vi "SMO.UI.ByRefWithEvents.TestLauncher.vi"() -> ()   [LabVIEW 2013, in "SMO.UI.ByRefWithEvents.lvclass"]
doc: "JKI State Machine Objects (SMO) 1.0.0.5\nJKI - JKI\nCopyright (c) 2016, JKI"
uses:
  SMO.UI.ByRefWithEvents.lvclass
  <vilib>/JKI/JKI SMO/SMO/SMO.lvclass
  <vilib>/JKI/JKI SMO/SMO.UI/SMO.UI.lvclass
panel:
  in  "Send":bool
  in  "Data":string
  out "error out":errorcluster
  in  "Stop":bool
  # "SMO UI Test Launcher"
  # "For instructions on how to use the JKI State Machine Objects, examples and video tutorials, visit:\nhttp://jki.net/state-machine-objects/\n\nJKI State Machine Objects™\nhttp://jki.net/state-machine-objects/\nCopyright (C) 2005-2015, JKI <info@jki.net>\nALL RIGHTS RESERVED"
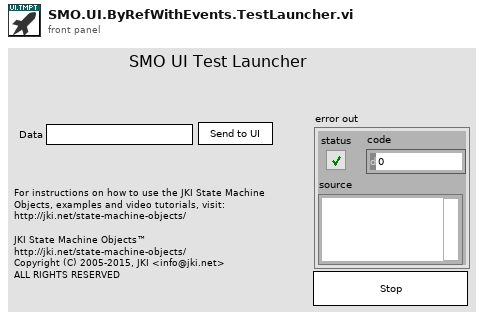
[diagram p1: front panel]
types:
  T1 = typedef "SMO.UI.lvclass/PublicEvents--Cluster.ctl" = cluster{"UI Hidden":refnum<user-event>, "UI State":refnum<user-event>}
  T2 = cluster{"SMO.Template Public Events":refnum<event-registration>, "Event Registration Refnum":refnum<event-registration>}
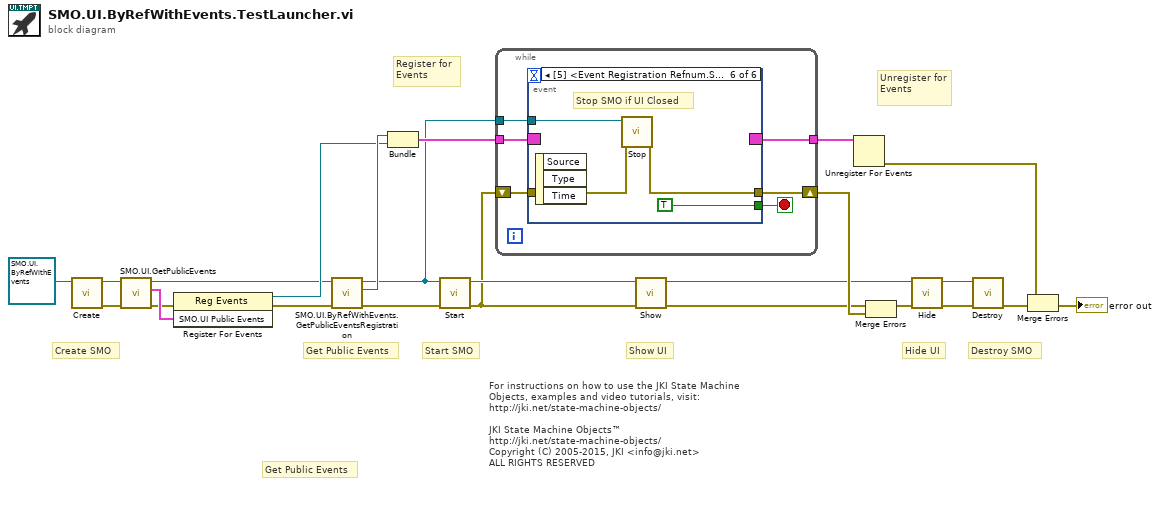
[diagram p0: block diagram]
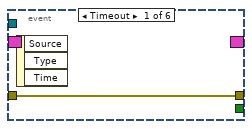
[diagram p2: hidden frame]
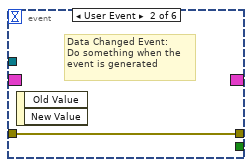
[diagram p3: hidden frame]
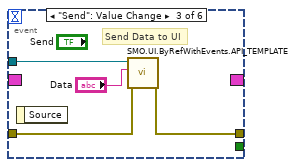
[diagram p4: hidden frame]
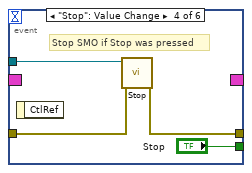
[diagram p5: hidden frame]
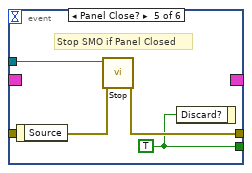
[diagram p6: hidden frame]
diagram:
  # "Get Public Events"
  # "Hide UI"
  # "Show UI"
  # "For instructions on how to use the JKI State Machine Objects, examples and video tutorials, visit:\nhttp://jki.net/state-machine-objects/\n\nJKI State Machine Objects™\nhttp://jki.net/state-machine-objects/\nCopyright (C) 2005-2015, JKI <info@jki.net>\nALL RIGHTS RESERVED"
  # "Get Public Events"
  # "Start SMO"
  # "Destroy SMO"
  # "Create SMO"
  # "Unregister for Events"
  # "Register for Events"
  n1 = call <vilib>:"Create.vi"("SMO"=refnum<class "SMO.UI.ByRefWithEvents.lvclass"> refnum ("SMO.Template.lvclass")) -> ("error out"=w2:errorcluster, "SMO out"=w5:refnum<class "SMO.UI.ByRefWithEvents.lvclass">)  [unwired: 8 in, 1 out]
  n2 = call <vilib>:"SMO.UI.GetPublicEvents.vi"("error in (no error)"=w2, "SMO.UI"=w5) -> ("error out"=w6:errorcluster, "SMO.UI Public Events"=w7:T1, "SMO.UI out"=w3:refnum<class "SMO.UI.ByRefWithEvents.lvclass">)  [unwired: 7 in]
  n3 = register-events(error in=w6, w7) -> (reference out=w4:refnum<event-registration>, error out=w1:errorcluster)  [unwired: 1 in]
  n4 = call "SMO.UI.ByRefWithEvents.GetPublicEventsRegistration.vi"("error in (no error)"=w1, "SMO.UI.ByRefWithEvents"=w3) -> ("error out"=w17:errorcluster, "SMO.Template Public Events"=w16:refnum<event-registration>, "SMO.UI.ByRefWithEvents out"=w15:refnum<class "SMO.UI.ByRefWithEvents.lvclass">)  [unwired: 7 in]
  n5 = Bundle("SMO.Template Public Events"=w16, "Event Registration Refnum"=w4) -> (w23:T2)  [unwired: 1 in]
  n6 = call <vilib>:"Start.vi"("error in (no error)"=w17, "SMO"=w15) -> ("error out"=w13:errorcluster, "SMO out"=w14:refnum<class "SMO.UI.ByRefWithEvents.lvclass">)  [unwired: 8 in]
  n7 = while {
    shift-right: [w29] -> w22
    shift-left: w13 -> [w28]
    tunnel: w23 -> [w27]
    tunnel: [w26] -> w24
    tunnel: w15 -> [w25]
    stop <- w30 stop-if-true
    n8 = event shown="[5] <Event Registration Refnum.SMO.UI Public Events.UI Hidden>: User Event" {
      selector: w27 -> [_ _ _ _ _ _]
      dyn-events: [_ _ _ _ _ _] -> w26
      timeout: _ -> [_ _ _ _ _ _]
      tunnel: [_ _ _ "Stop" w41 TRUE ("OK")] -> w30
      tunnel: w25 -> [_ _ w36 w38 w44 w48]
      tunnel: [w31 w32 w33 w39 w43 w47] -> w29
      tunnel: w28 -> [w31 w32 w34 w37 w42 w46]
      event Timeout {
        n9 = event-data() -> ()  [unwired: 1 in, 3 out]
      }
      event User Event {
        # "Data Changed Event:\nDo something when the\nevent is generated"
        n10 = event-data() -> ()  [unwired: 1 in, 2 out]
      }
      event "Send": Value Change {
        # "Send Data to UI"
        n11 = event-data() -> ()  [unwired: 1 in, 1 out]
        n12 = call "SMO.UI.ByRefWithEvents.API_TEMPLATE.vi"("error in (no error)"=w34, "myData"="Data", "SMO.UI.ByRefWithEvents"=w36) -> ("error out"=w33:errorcluster)  [unwired: 6 in, 2 out]
      }
      event "Stop": Value Change {
        # "Stop SMO if Stop was pressed"
        n13 = event-data() -> ()  [unwired: 1 in, 1 out]
        n14 = call <vilib>:"Stop.vi"("error in (no error)"=w37, "SMO"=w38) -> ("error out"=w39:errorcluster)  [unwired: 8 in, 1 out]
      }
      event Panel Close? {
        w41 = TRUE ("OK")
        # "Stop SMO if Panel Closed"
        n15 = event-data() -> ()  [unwired: 1 in, 1 out]
        n16 = call <vilib>:"Stop.vi"("error in (no error)"=w42, "SMO"=w44) -> ("error out"=w43:errorcluster)  [unwired: 8 in, 1 out]
        n17 = event-data("Discard?"=w41) -> ()  [unwired: 1 in, 1 out]
      }
      event User Event {
        # "Stop SMO if UI Closed"
        n18 = event-data() -> ()  [unwired: 1 in, 3 out]
        n19 = call <vilib>:"Stop.vi"("error in (no error)"=w46, "SMO"=w48) -> ("error out"=w47:errorcluster)  [unwired: 8 in, 1 out]
      }
    }
  }
  n20 = call <vilib>:"Show.vi"("error in (no error)"=w13, "SMO.UI"=w14) -> ("error out"=w12:errorcluster, "SMO.UI out"=w11:refnum<class "SMO.UI.ByRefWithEvents.lvclass">)  [unwired: 8 in]
  n21 = Unregister For Events(event registration refnum=w24) -> (error out=w21:errorcluster)  [unwired: 1 in]
  n22 = Merge Errors(w12, w22) -> (w9:errorcluster)
  n23 = call <vilib>:"Hide.vi"("error in (no error)"=w9, "SMO.UI"=w11) -> ("error out"=w8:errorcluster, "SMO.UI out"=w10:refnum<class "SMO.UI.ByRefWithEvents.lvclass">)  [unwired: 8 in]
  n24 = call <vilib>:"Destroy.vi"("error in (no error)"=w8, "SMO"=w10) -> ("error out"=w19:errorcluster)  [unwired: 9 in]
  n25 = Merge Errors(w21, w19) -> (→"error out":errorcluster)
